vi "ControlTemperatura.vi"(0 "Chassis Temperature":i16) -> (1 "Aviso temperatura":string, 2 "Boolean":bool, 3 "T fuera rango":bool)   [LabVIEW 2015]
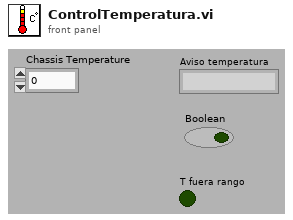
[diagram p1: front panel]
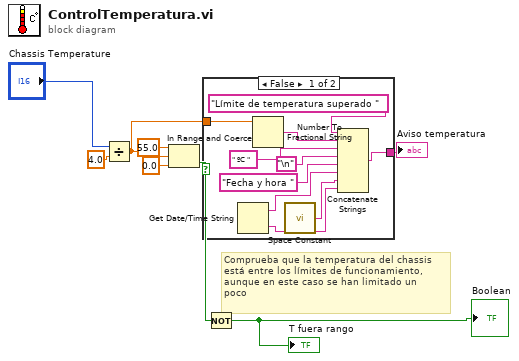
[diagram p0: block diagram]
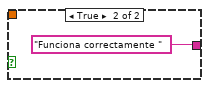
[diagram p2: hidden frame]
diagram:
  # "Comprueba que la temperatura del chassis\nestá entre los límites de funcionamiento,\naunque en este caso se han limitado un \npoco"
  n1 = Divide(x="Chassis Temperature", y=4.0) -> (x/y=w8:dbl)
  n2 = In Range and Coerce(upper limit=55.0, x=w8, lower limit=0.0) -> (In Range?=w1:bool)  [unwired: 1 out]
  n3 = case shown="False" w1 {
    tunnel: w8 -> [w12 _]
    tunnel: [w11 "Funciona correctamente " ("String")] -> w6
    frame False {
      n4 = Get Date/Time String() -> (date string=w15:string, time string=w13:string)  [unwired: 3 out]
      n5 = Number To Fractional String(number=w12) -> (F-format string=w17:string)  [unwired: 3 out]
      n6 = call <vilib>:"Space Constant.vi"() -> ("String"=w14:string)
      n7 = Concatenate Strings("Límite de temperatura superado ", w17, " ºC ", "\n", "Fecha y hora ", w15, w14, w13) -> (w11:string)
    }
    frame True {
    }
  }
  "Aviso temperatura" <- w6
  n8 = Not(x=w1) -> (.not. x?=→"T fuera rango" →"Boolean":bool)
